vi "Globals.vi"() -> ()   [LabVIEW 2019, in "RT_Game.lvlib"]
uses:
  RT_Game.lvlib
panel:
  out "CameraMoving?":bool
  in  "volume_effects":dbl=0.2
  in  "volume_music":dbl=0.2
  in  "deltaT":dbl
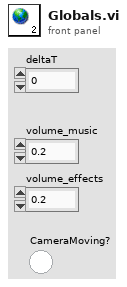
[diagram p1: front panel]
diagram:
